vi "UI.vi"(7 "Consumer Data":T1, 8 "error in (no error)":errorcluster, 9 "function name":string, 11 "session in":refnum<k35>) -> (0 "error out":errorcluster, 3 "session out":refnum<k35>)   [LabVIEW 2018]
uses:
  Consumer_Data.ctl
  enumsUI.ctl
panel:
  in  "Emergency Stop":bool
  in  "Trigger":bool=TRUE
  in  "Table Control":string[][](table)
  in  "Back":bool
  in  "Update":bool
  # "UPDATE THRESHOLDS"
  # "BACK"
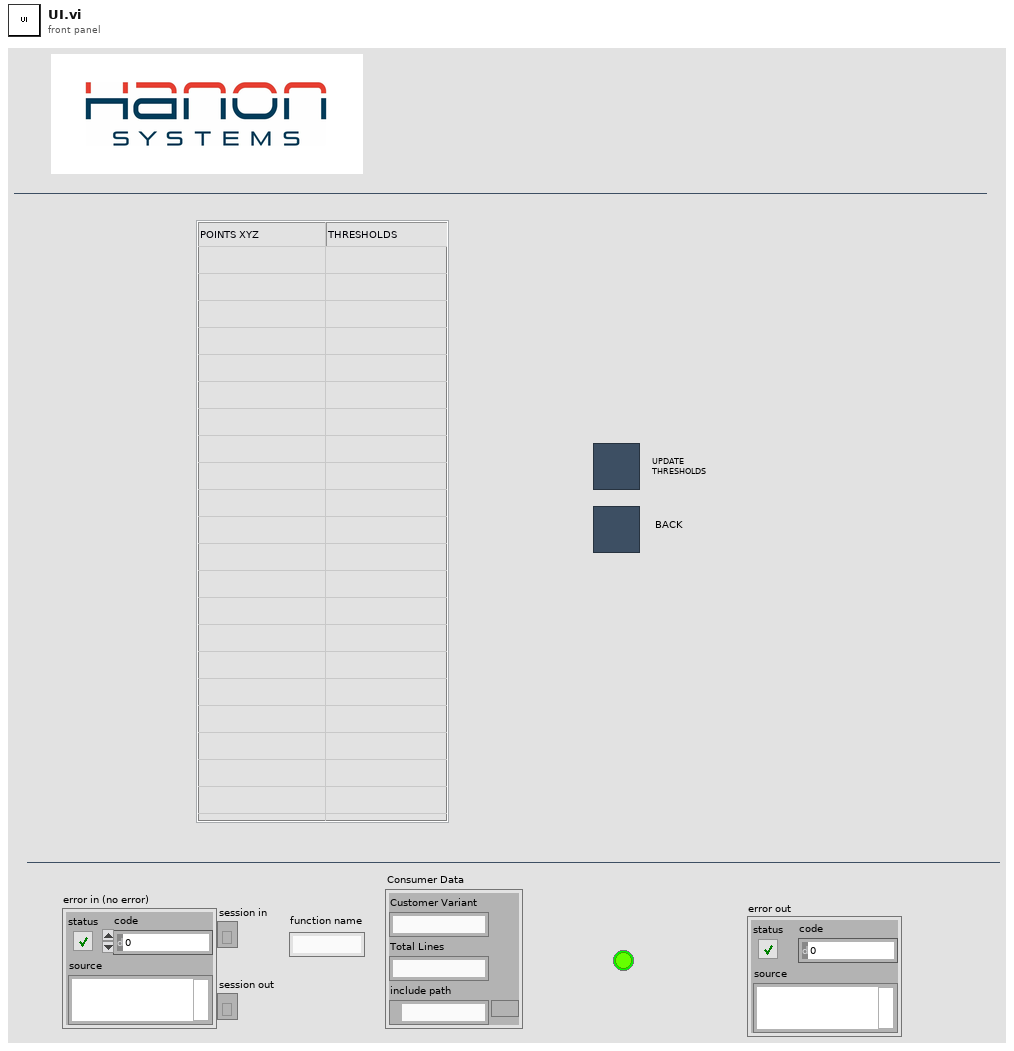
[diagram p1: front panel]
types:
  T1 = typedef "Consumer_Data.ctl" = cluster{"Customer Variant":string, "Total Lines":string, "include path":path}
  T2 = typedef "enumsUI.ctl" = enum16{"Timeout", "Table Refresh", "Update", "Exit"}
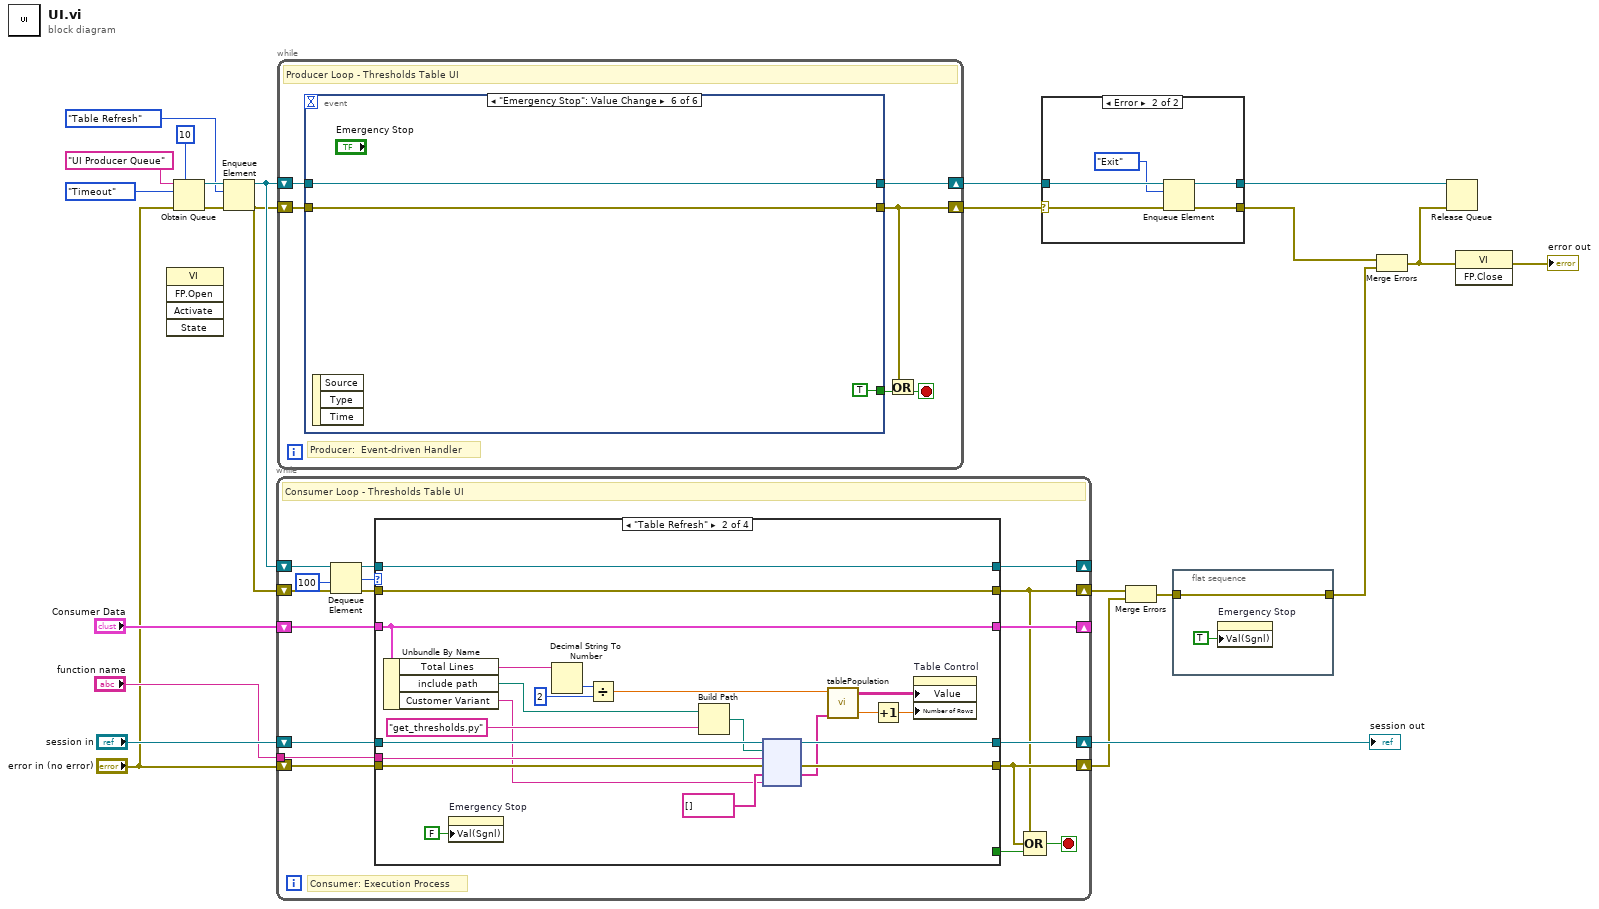
[diagram p0: block diagram]
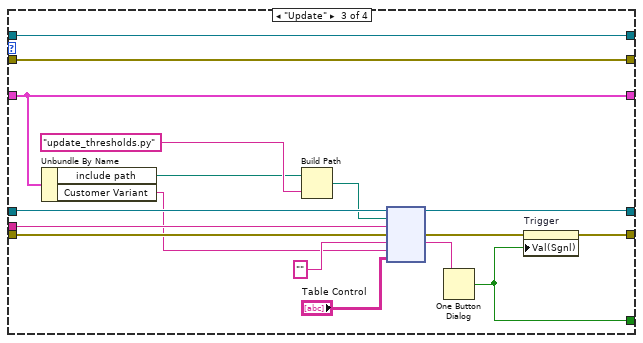
[diagram p4: hidden frame]
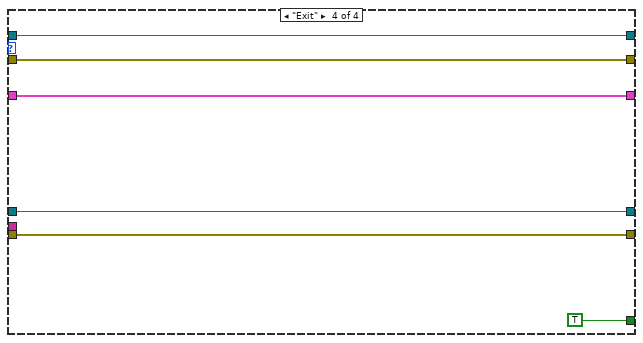
[diagram p5: hidden frame]
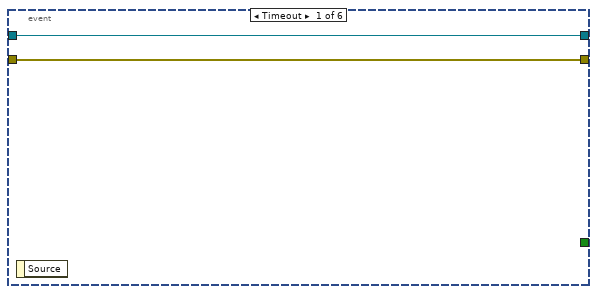
[diagram p6: hidden frame]
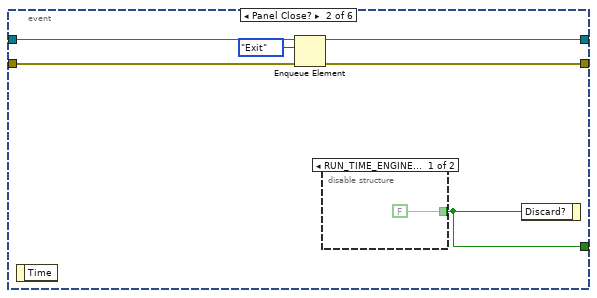
[diagram p7: hidden frame]
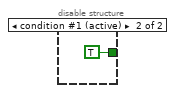
[diagram p8: hidden frame]
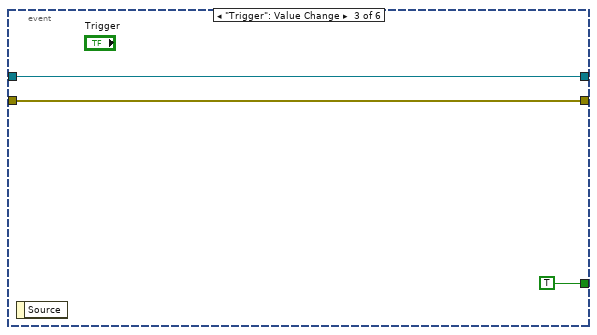
[diagram p9: hidden frame]
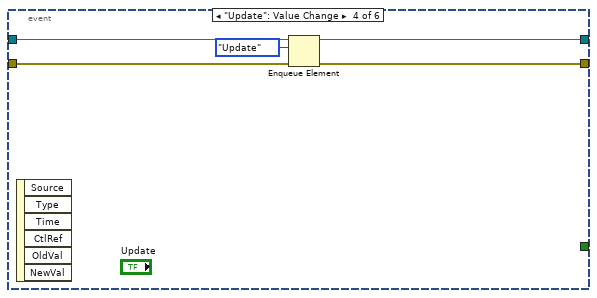
[diagram p10: hidden frame]
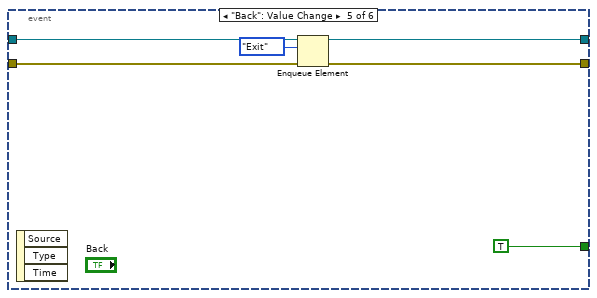
[diagram p11: hidden frame]
diagram:
  n1 = invoke class="VI" method="FP.Open"() -> ()  [unwired: 5 in, 5 out]
  n2 = Obtain Queue(max queue size (-1, unlimited)=10, name (unnamed)="UI Producer Queue", element data type=enumsUI."Timeout", error in (no error)="error in (no error)") -> (queue out=w17:refnum<queue>, error out=w15:errorcluster)  [unwired: 1 in, 1 out]
  n3 = Enqueue Element(queue=w17, element=enumsUI."Table Refresh", error in (no error)=w15) -> (queue out=w16:refnum<queue>, error out=w14:errorcluster)  [unwired: 1 in, 1 out]
  n4 = while {
    shift-right: [w25] -> w3
    shift-left: "error in (no error)" -> [w40]
    shift-right: [w24] -> w4
    shift-left: w14 -> [w39]
    shift-right: [w35] -> _
    shift-left: w16 -> [w37]
    shift-right: [w32] -> w20
    shift-left: "session in" -> [w31]
    tunnel: "function name" -> [w30]
    shift-right: [w28] -> _
    shift-left: "Consumer Data" -> [w29]
    stop <- w26 stop-if-true
    # "Consumer: Execution Process"
    # "Consumer Loop - Thresholds Table UI"
    n5 = Dequeue Element(queue=w37, timeout in ms (-1)=100, error in (no error)=w39) -> (queue out=w36:refnum<queue>, element=w34:T2, error out=w38:errorcluster)  [unwired: 1 out]
    n6 = case shown="\"Table Refresh\"" w34 {
      tunnel: w40 -> [w45 w63 w80 w90]
      tunnel: [w45 w62 w70 w90] -> w25
      tunnel: [w44 w67 w83 w89] -> w24
      tunnel: w38 -> [w44 w67 w83 w89]
      tunnel: w36 -> [w43 w66 w84 w88]
      tunnel: [w43 w66 w84 w88] -> w35
      tunnel: [w42 w64 w81 w87] -> w32
      tunnel: w31 -> [w42 w65 w82 w87]
      tunnel: [_ _ w69 TRUE] -> w27
      tunnel: w30 -> [_ w61 w78 _]
      tunnel: [w41 w53 w74 w85] -> w28
      tunnel: w29 -> [w41 w53 w74 w85]
      frame "Timeout", Default {
      }
      frame "Table Refresh" {
        n7 = Unbundle By Name(w53) -> ("Total Lines"=w50:string, "include path"=w48:path, "Customer Variant"=w47:string)
        n8 = property on="Emergency Stop" class="Bool"("Val(Sgnl)"=FALSE ("Value (Signaling)")) -> ()  [unwired: 2 in, 2 out]
        n9 = Decimal String To Number(string=w50) -> (number=w52:i32)  [unwired: 2 in, 1 out]
        n10 = Divide(x=w52, y=2) -> (x/y=w49:dbl)
        n11 = Build Path(base path=w48, name or relative path="get_thresholds.py") -> (appended path=w58:path)
        n12 = node(w65, w58, w61, w63, string[] [], w47) -> (w64:refnum<k35>, w62:errorcluster, w57:string[])  [unwired: 1 in, 2 out]
        n13 = call "tablePopulation.vi"("new element/subarray"=w57, "Numeric"=w49) -> ("Numeric 2"=w56:dbl, "output array"=w54:string[][])  [unwired: 7 in, 1 out]
        n14 = Increment(x=w56) -> (x+1=w55:dbl)
        n15 = property on="Table Control" class="Tbl (strict)"("Value"=w54, "Number of Rows"=w55) -> ()  [unwired: 2 in, 2 out]
      }
      frame "Update" {
        n16 = Unbundle By Name(w74) -> ("include path"=w73:path, "Customer Variant"=w72:string)
        n17 = Build Path(base path=w73, name or relative path="update_thresholds.py") -> (appended path=w76:path)
        n18 = node(w82, w76, w78, w80, "", w72, "Table Control") -> (w81:refnum<k35>, w71:errorcluster, w68:string)  [unwired: 2 in, 2 out]
        n19 = One Button Dialog(message=w68) -> (true=w69:bool)  [unwired: 1 in]
        n20 = property on="Trigger" class="Bool (strict)"(error in=w71, "Val(Sgnl)"=w69) -> (error out=w70:errorcluster)  [unwired: 1 in, 1 out]
      }
      frame "Exit" {
        (unwired) TRUE
      }
    }
    n21 = Compound Arithmetic op=OR(w24, w25, w27) -> (w26:bool)
  }
  "session out" <- w20
  n22 = while {
    shift-right: [w94] -> w9
    shift-left: w16 -> [w95]
    shift-right: [w91] -> w7
    shift-left: w14 -> [w96]
    stop <- w92 stop-if-true
    # "Producer:  Event-driven Handler"
    # "Producer Loop - Thresholds Table UI"
    n23 = event shown="[5] \"Emergency Stop\": Value Change" {
      selector: _ -> [_ _ _ _ _ _]
      dyn-events: _ -> [_ _ _ _ _ _]
      timeout: _ -> [_ _ _ _ _ _]
      tunnel: [w98 w102 w109 w114 w119 w123] -> w94
      tunnel: w96 -> [w97 w101 w108 w113 w117 w122]
      tunnel: [w97 w100 w108 w112 w118 w122] -> w91
      tunnel: w95 -> [w98 w103 w109 w111 w120 w123]
      tunnel: [_ w104 TRUE _ TRUE TRUE] -> w93
      event Timeout {
        n24 = event-data() -> ()  [unwired: 1 in, 1 out]
      }
      event Panel Close? {
        n25 = event-data() -> ()  [unwired: 1 in, 1 out]
        n26 = Enqueue Element(queue=w103, element=enumsUI."Exit", error in (no error)=w101) -> (queue out=w102:refnum<queue>, error out=w100:errorcluster)  [unwired: 1 in, 1 out]
        n27 = disable-structure shown="RUN_TIME_ENGINE==True" {
          disable-tunnel: [FALSE TRUE] -> w104
          frame condition #0 {
          }
          frame condition #1 (active) {
          }
        }
        n28 = event-data("Discard?"=w104) -> ()  [unwired: 1 in, 1 out]
      }
      event "Trigger": Value Change {
        n29 = event-data() -> ()  [unwired: 1 in, 1 out]
      }
      event "Update": Value Change {
        n30 = event-data() -> ()  [unwired: 1 in, 6 out]
        n31 = Enqueue Element(queue=w111, element=enumsUI."Update", error in (no error)=w113) -> (queue out=w114:refnum<queue>, error out=w112:errorcluster)  [unwired: 1 in, 1 out]
      }
      event "Back": Value Change {
        n32 = event-data() -> ()  [unwired: 1 in, 3 out]
        n33 = Enqueue Element(queue=w120, element=enumsUI."Exit", error in (no error)=w117) -> (queue out=w119:refnum<queue>, error out=w118:errorcluster)  [unwired: 1 in, 1 out]
      }
      event "Emergency Stop": Value Change {
        n34 = event-data() -> ()  [unwired: 1 in, 3 out]
      }
    }
    n35 = Or(x=w91, y=w93) -> (x .or. y?=w92:bool)
  }
  n36 = case shown="Error" w7 {
    selector: w7 -> [w124 w130]
    tunnel: w9 -> [w125 w129]
    tunnel: [w125 w128] -> w8
    tunnel: [w124 w127] -> w6
    frame No Error {
    }
    frame Error {
      n37 = Enqueue Element(queue=w129, element=enumsUI."Exit", error in (no error)=w130) -> (queue out=w128:refnum<queue>, error out=w127:errorcluster)  [unwired: 1 in, 1 out]
    }
  }
  n38 = Merge Errors(w4, w3) -> (w2:errorcluster)
  n39 = flat-sequence {
    tunnel: w2 -> [w131]
    tunnel: [w131] -> w1
    frame #0 {
      n40 = property on="Emergency Stop" class="Bool"("Val(Sgnl)"=TRUE ("Value (Signaling)")) -> ()  [unwired: 2 in, 2 out]
    }
  }
  n41 = Merge Errors(w6, w1) -> (w5:errorcluster)
  n42 = Release Queue(queue=w8, error in (no error)=w5) -> ()  [unwired: 1 in, 3 out]
  n43 = invoke class="VI" method="FP.Close"(error in=w5) -> (error out=→"error out":errorcluster)  [unwired: 2 in, 2 out]
